vi "探头模板-2-8.vi"() -> ()   [LabVIEW 2017]
uses:
  <vilib>/Utility/miscctls.llb/LVPoint32TypeDef.ctl
  <vilib>/Utility/miscctls.llb/LVPositionTypeDef.ctl
panel:
  in  "鼠标坐标":T1 caption="坐标"
  out "计算时间":dbl
  in  "坐标映射信号":bool=TRUE
  in  "停止":bool=TRUE
  out "探头地址":T2(ring)
  out "探头信息":string
  out "测量值":dbl format="%.2g"
  out "探头状态":T3(ring)=enum."一级报警"
  out "单位":enum16{"μSv/h", "mSv/h"}(ring)
  out "限值1":string="一级限值："
  out "限值2":string="二级限值："
  out "累积剂量":string="二级限值："
  in  "数据簇":T4
  out "数值":string
  in  "XY图":cluster{timestamp[], dbl[]}[](graph)
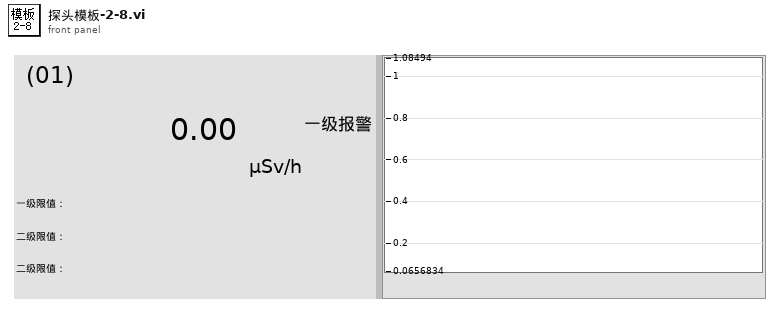
[diagram p1: front panel]
types:
  T1 = typedef "LVPoint32TypeDef.ctl" = cluster{"Horizontal":i32, "Vertical":i32}
  T2 = enum16{"(01)", "(02)", "(03)", "(04)", "(05)", "(06)", "(07)", "(08)", "(09)", "(10)", "(11)", "(12)", "(13)", "(14)", "(15)", "(16)", "(17)", "(18)", "(19)", "(20)", "(21)", "(22)", "(23)", "(24)", "(25)", "(26)", "(27)", "(28)", "(29)", "(30)", "(31)", "(32)", "(33)", "(34)", "(35)"}
  T3 = enum16{"正常", "未启用", "离线", "一级报警", "二级报警", "累积报警"}
  T4 = cluster{"启用状态？":bool, "测量值":cluster{"X":timestamp, "Y":dbl}, "限值簇":cluster{"限值1":dbl, "限值2":dbl, "探头限值":enum16{"一级限值", "二级限值"}}, "报警状态":enum16{"正常", "一级报警", "二级报警", "累积报警"}, "探头信息":string, "探头地址":i32, "累积剂量":cluster{"设备名称":string, "启用累积？":bool, "起始时间":timestamp, "累积剂量":dbl, "累积报警阈值":dbl}}
  T5 = cluster{"限值1":dbl, "限值2":dbl, "探头限值":enum16{"一级限值", "二级限值"}}
  T6 = typedef "LVPositionTypeDef.ctl" = cluster{"Left":i32, "Top":i32}
  T7 = cluster{"设备名称":string, "启用累积？":bool, "起始时间":timestamp, "累积剂量":dbl, "累积报警阈值":dbl}
  T8 = typedef "LVBoundsTypeDef.ctl" = cluster{"Width":u32, "Height":u32}
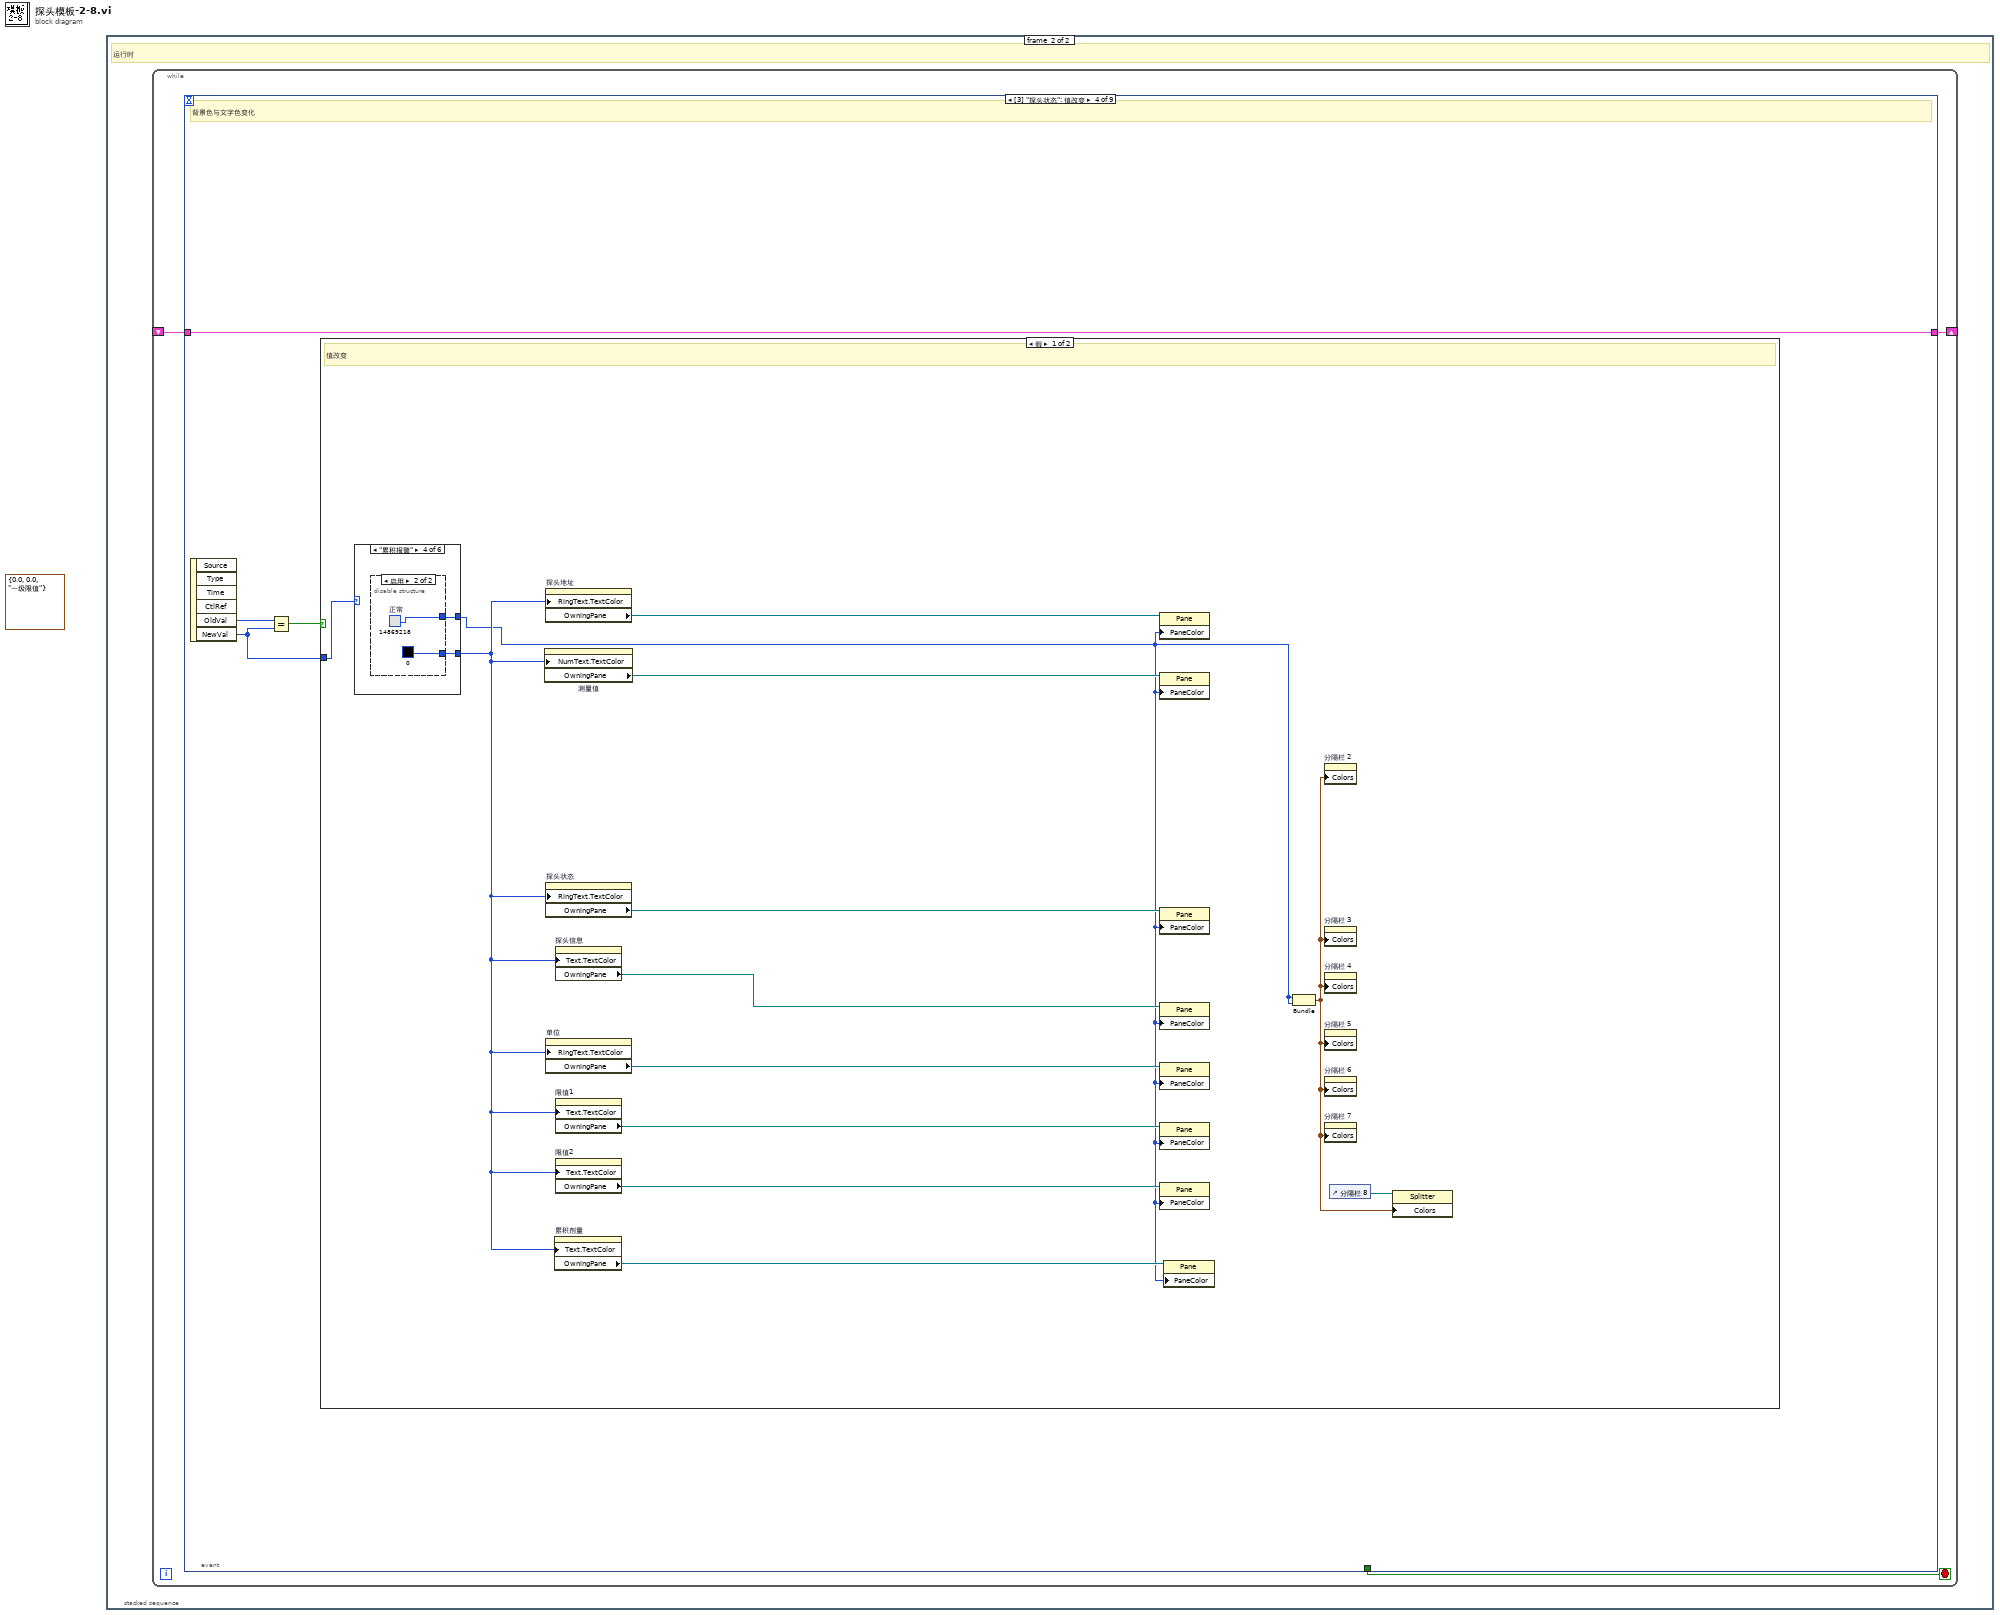
[diagram p0: block diagram]
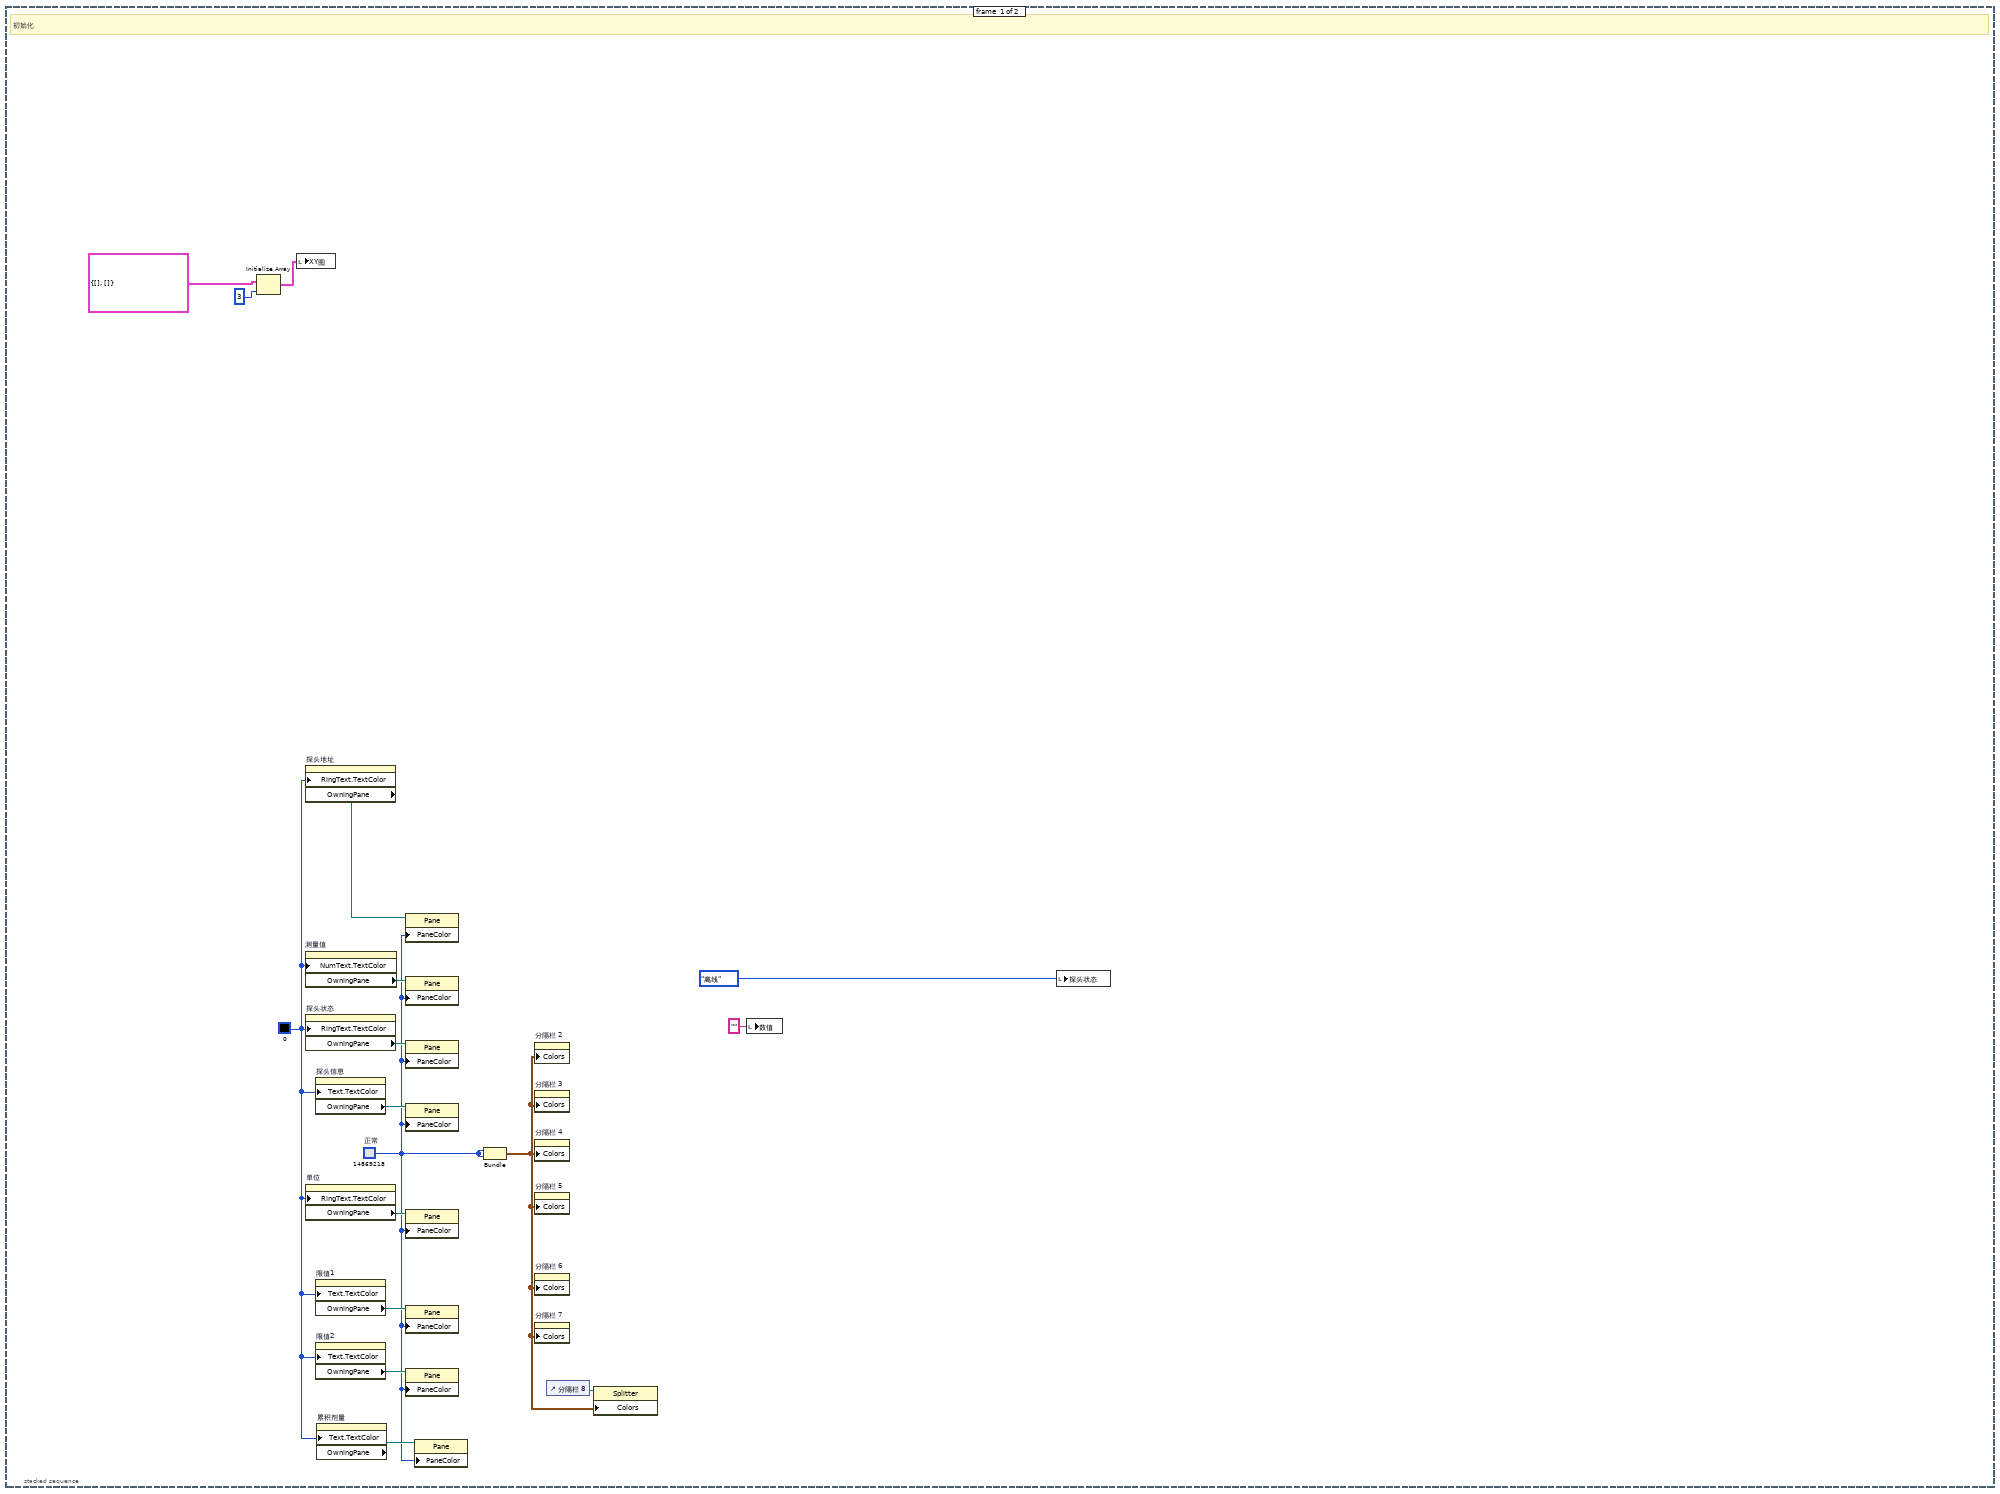
[diagram p2: hidden frame]
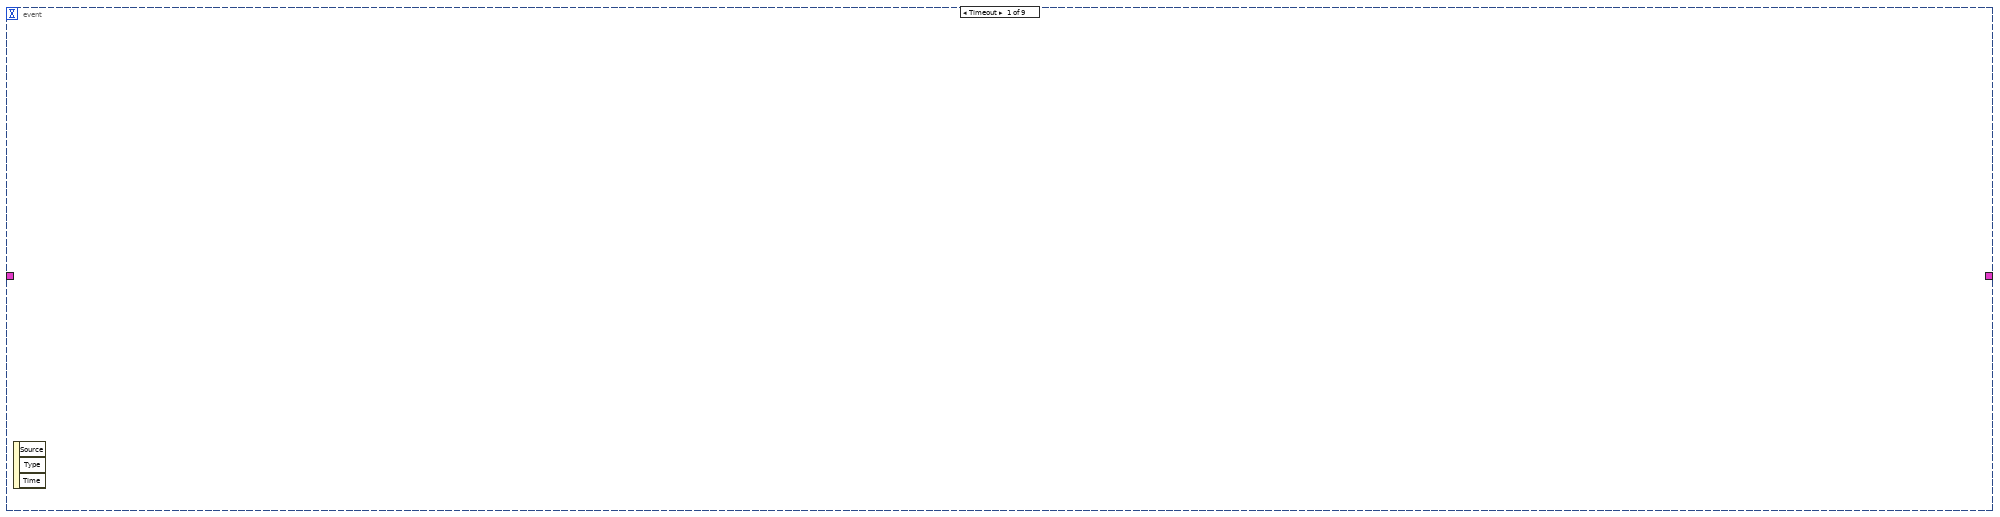
[diagram p3: hidden frame]
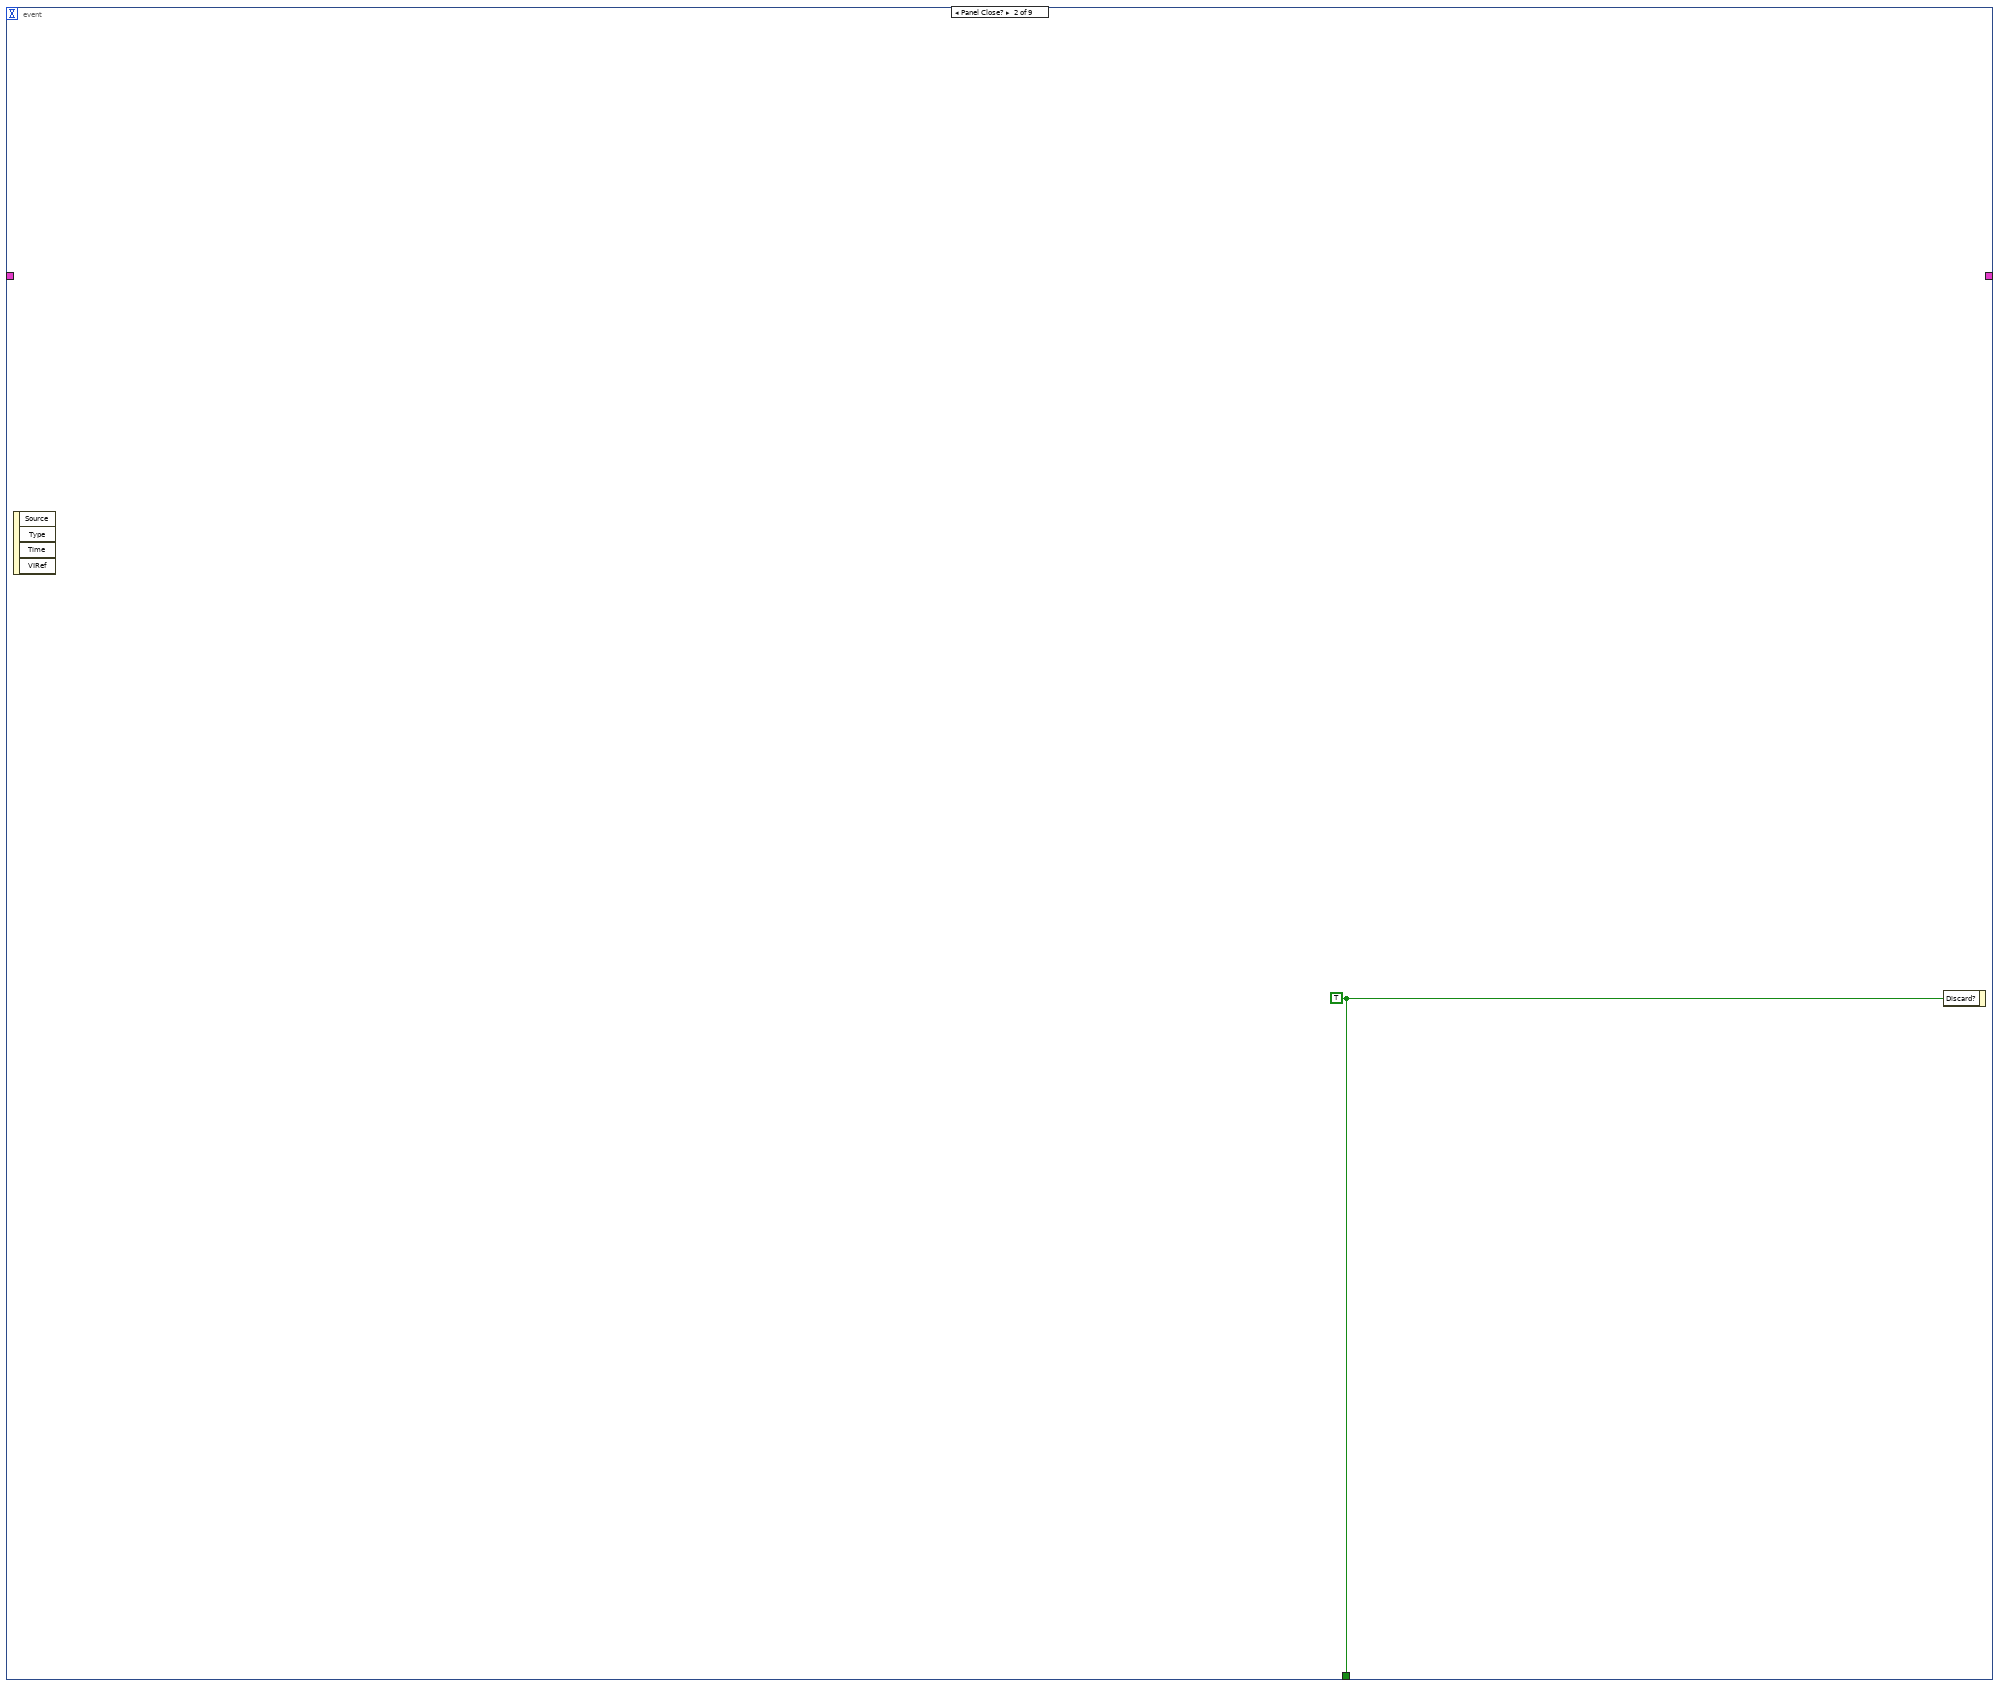
[diagram p4: hidden frame]
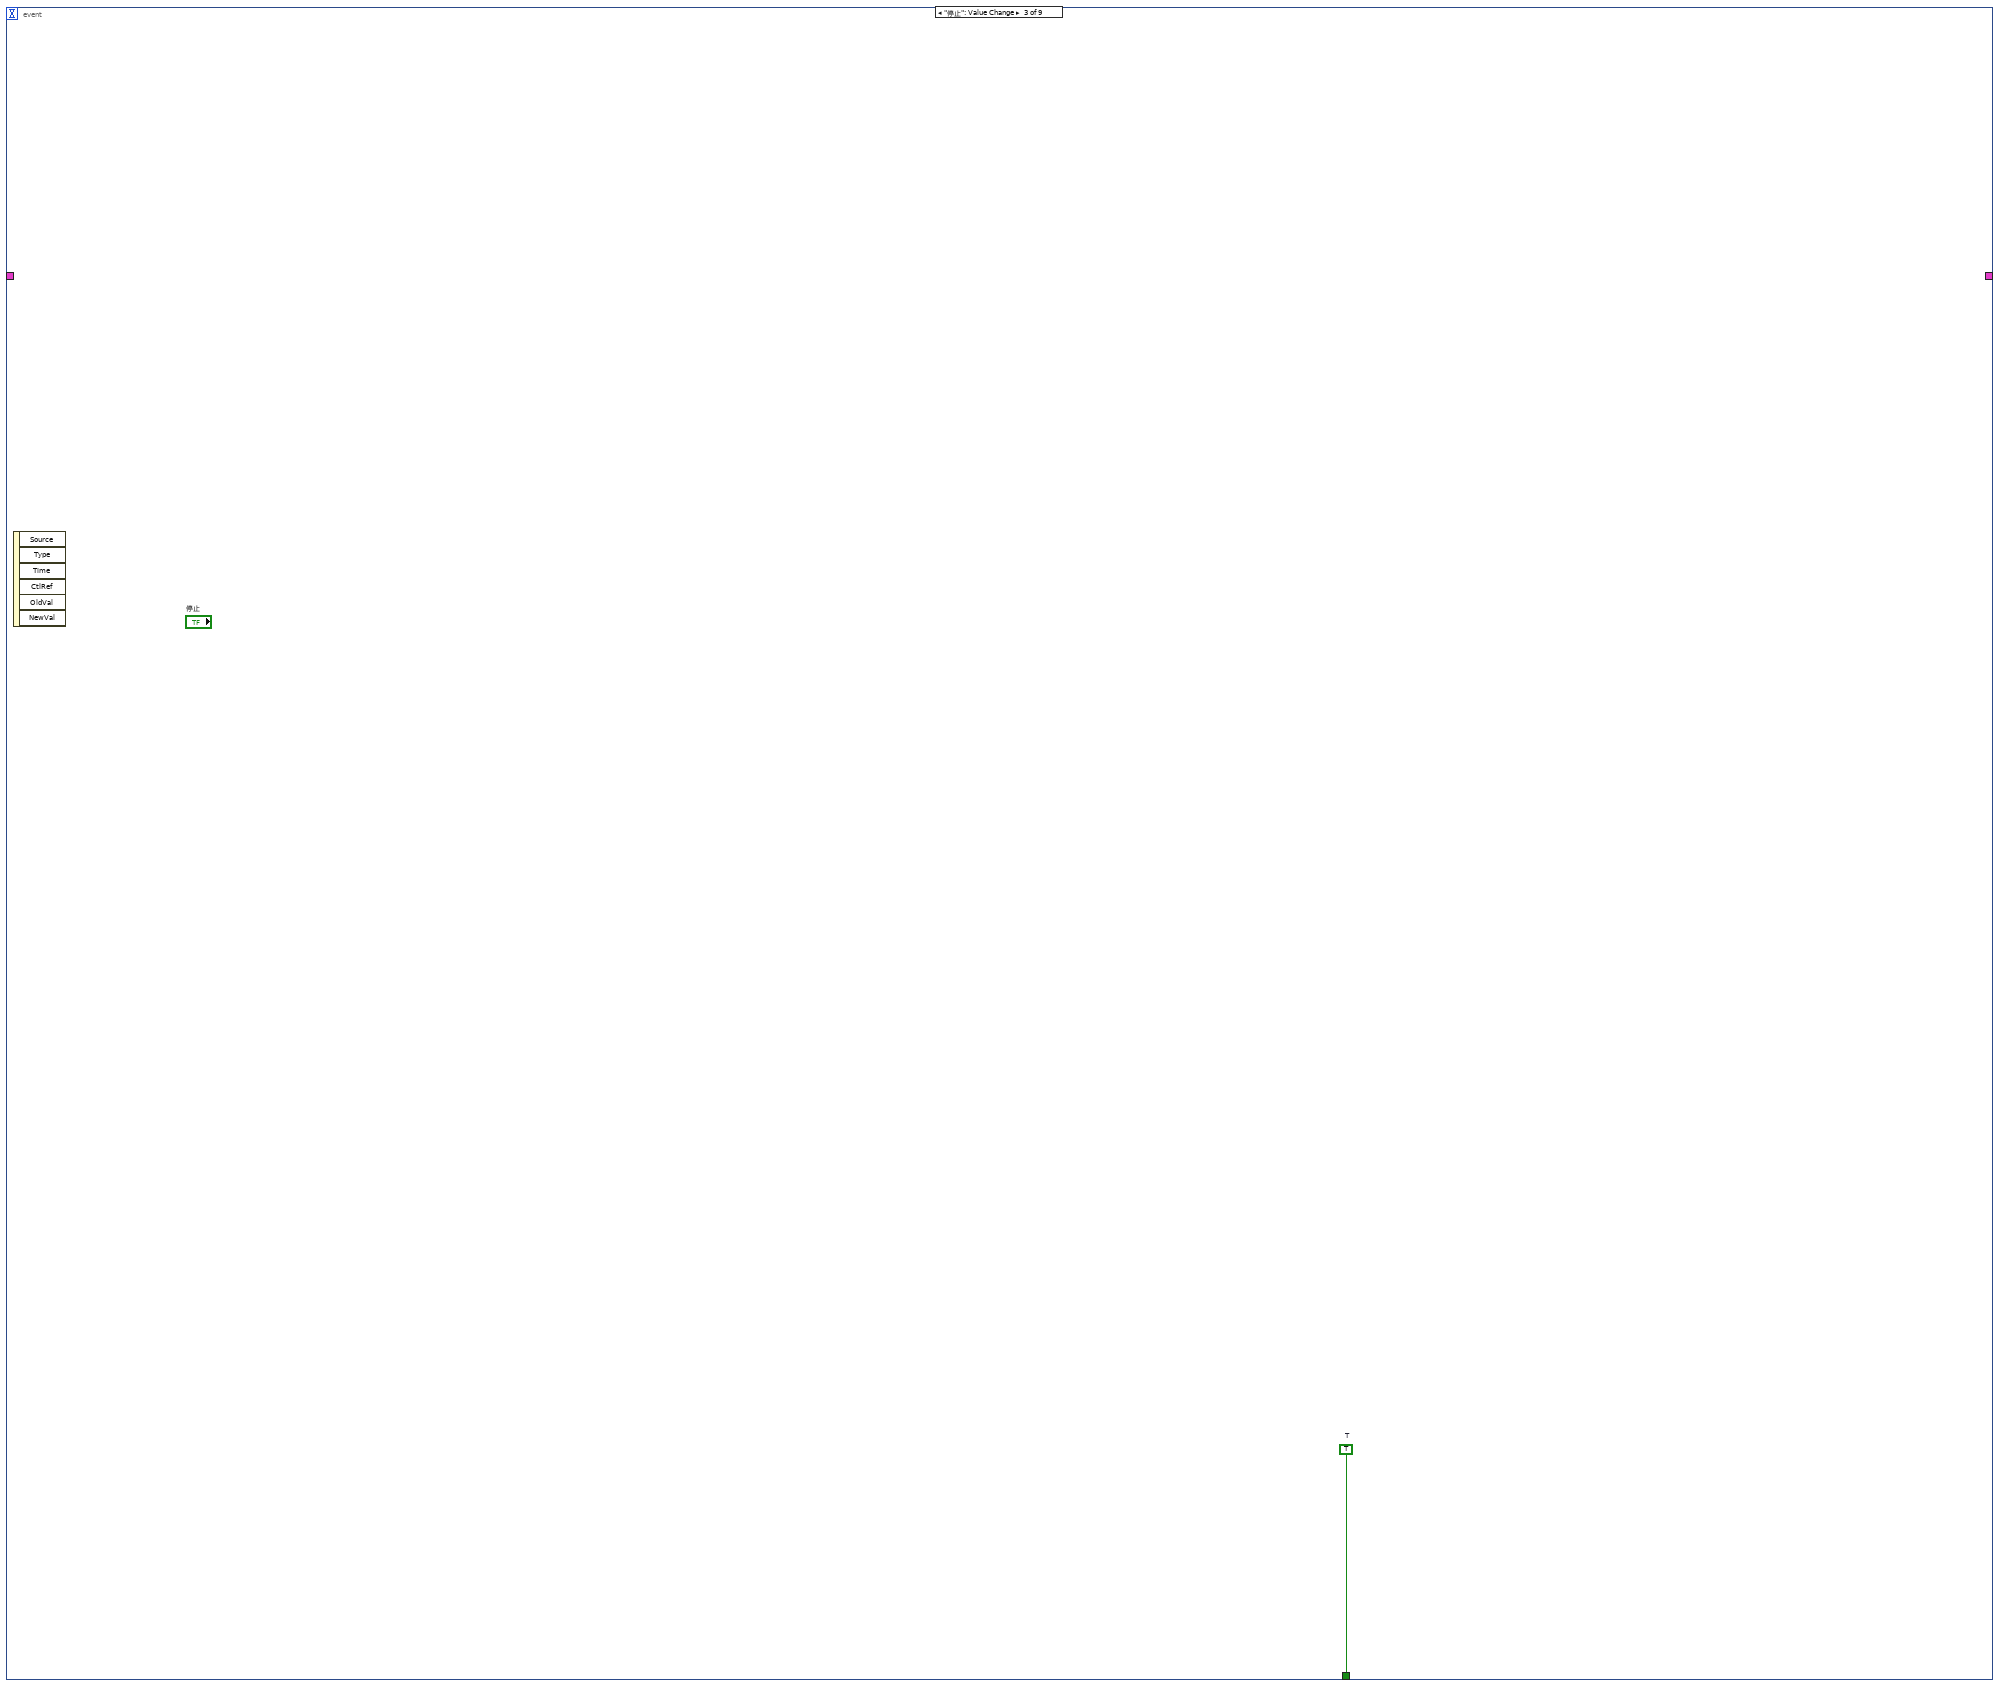
[diagram p5: hidden frame]
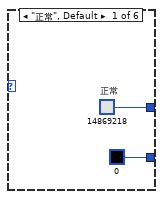
[diagram p6: hidden frame]
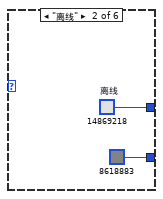
[diagram p7: hidden frame]
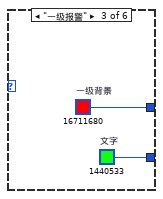
[diagram p8: hidden frame]
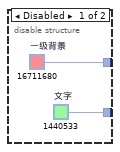
[diagram p9: hidden frame]
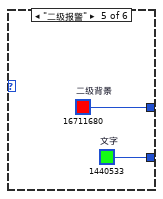
[diagram p10: hidden frame]
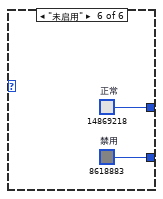
[diagram p11: hidden frame]
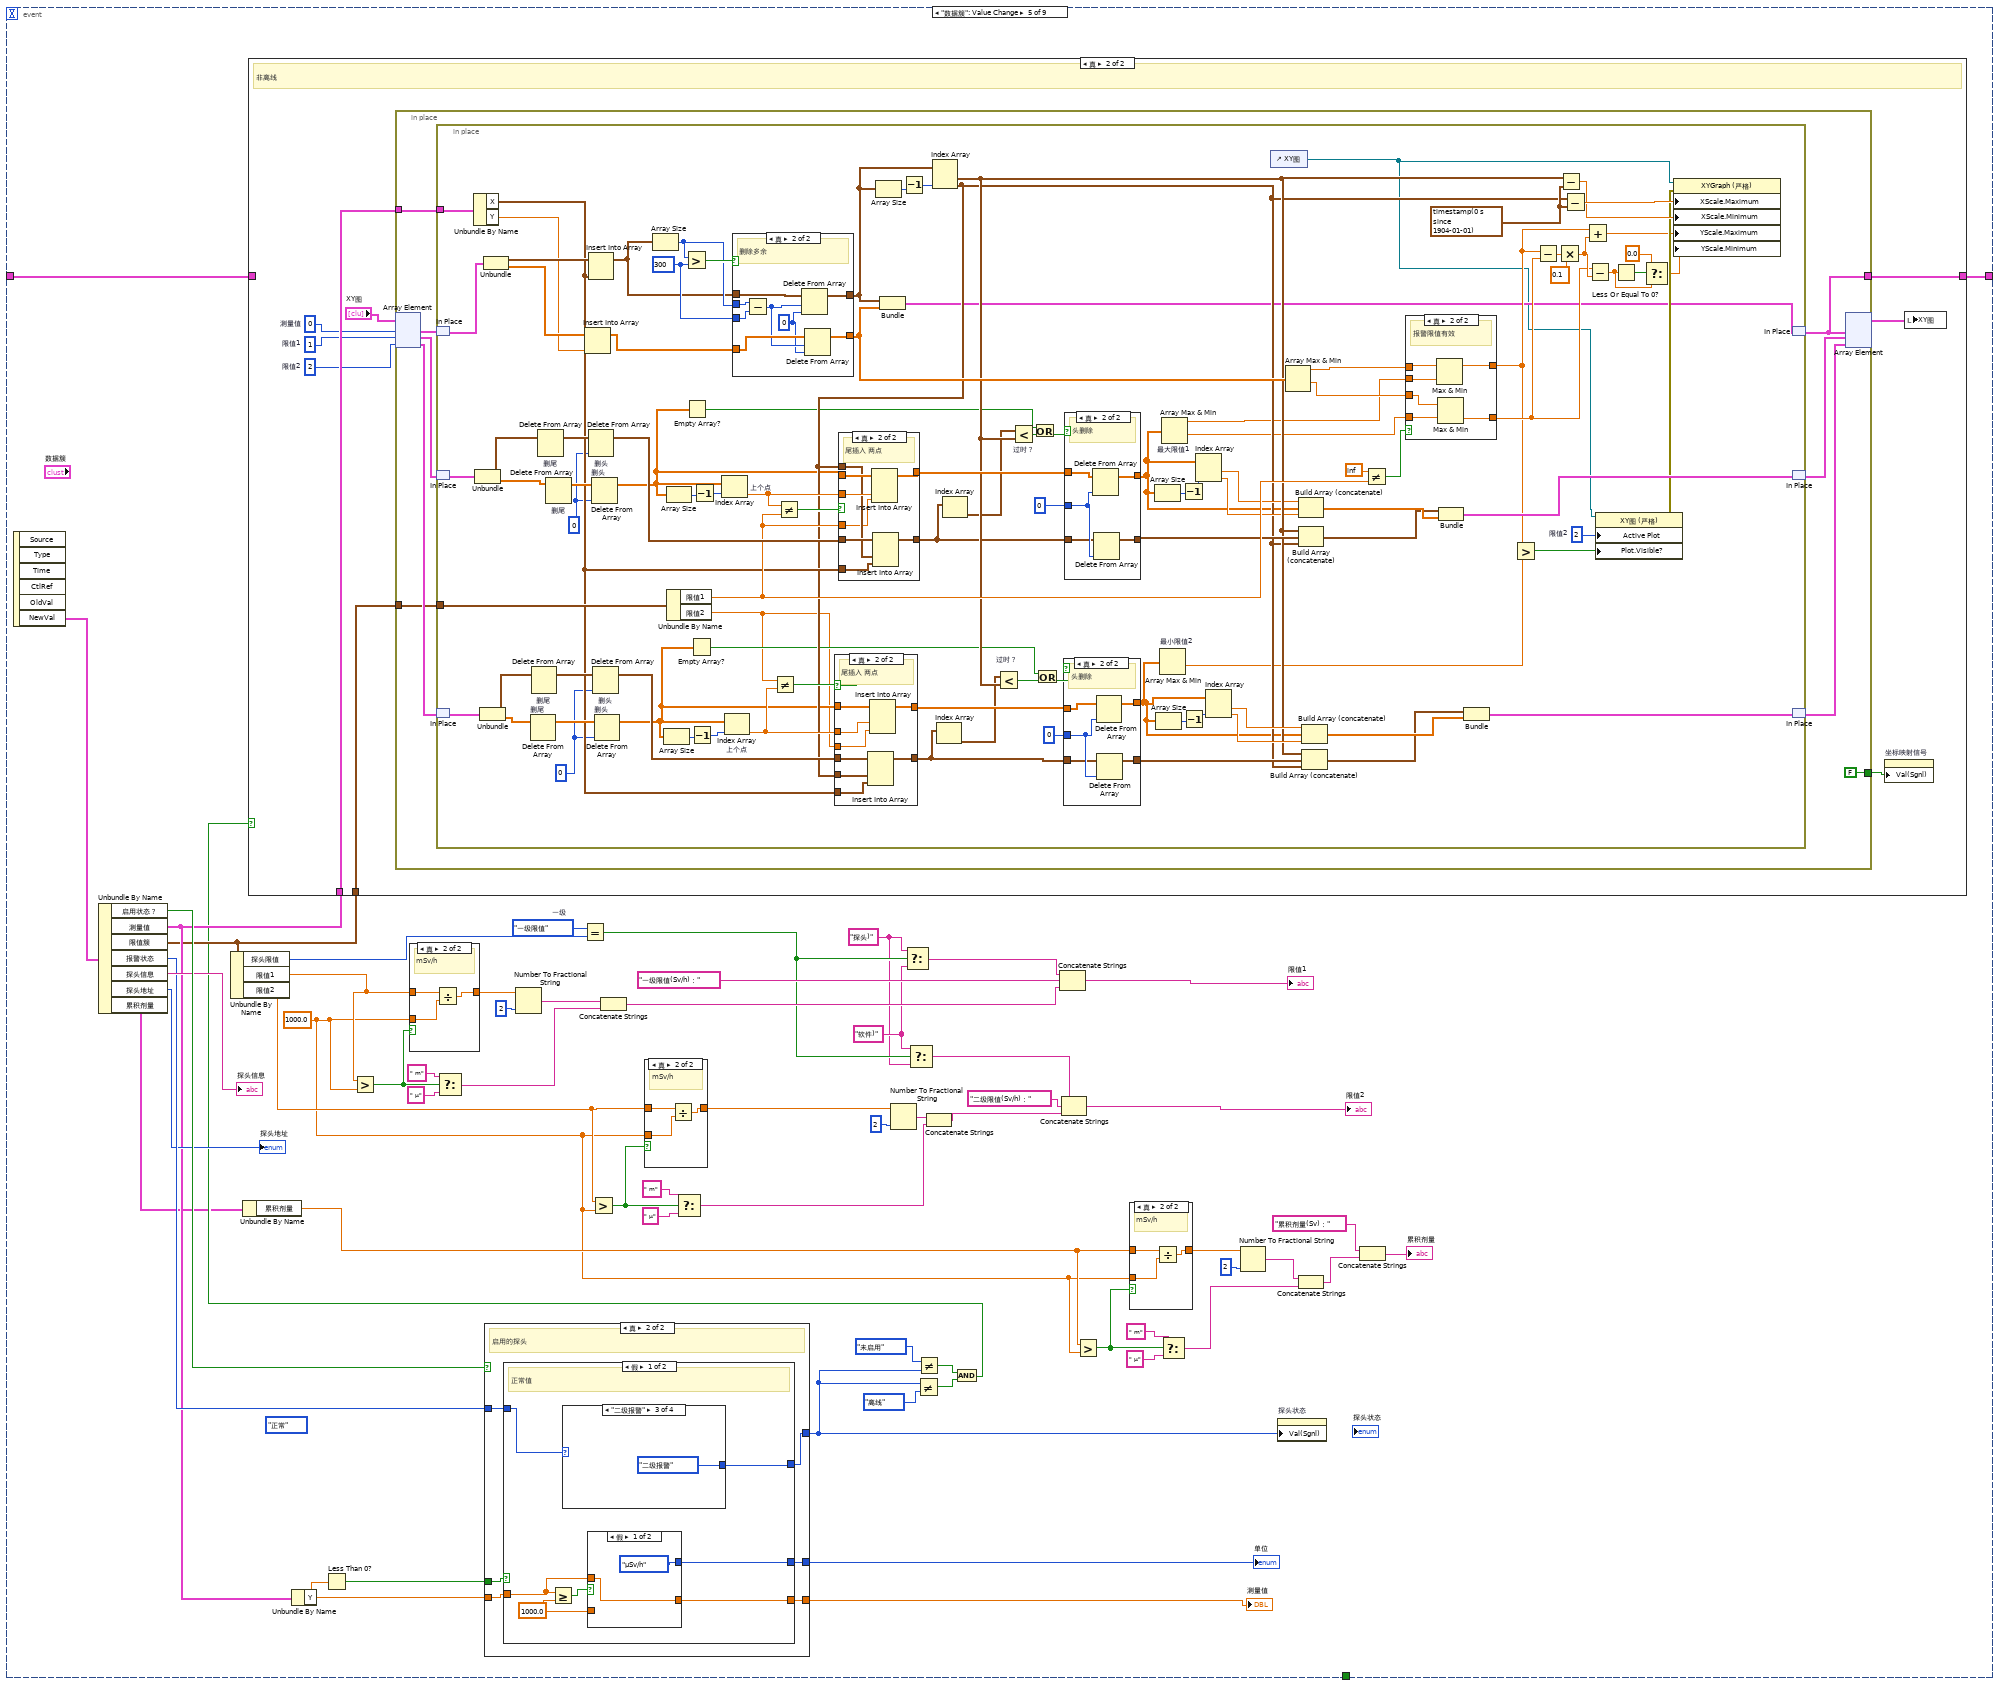
[diagram p13: hidden frame]
diagram:
  (unwired) T5 {"限值1"=0.0, "限值2"=0.0, "探头限值"=enum."一级限值"} ("探头限值簇")
  n1 = stacked-sequence {
    frame #0 {
      w3 = u32 0
      w2 = u32 14869218  # 正常
      # "初始化"
      n2 = Initialize Array(cluster{timestamp[], dbl[]} {[], []}, 3 ("维数大小")) -> (w7:cluster{timestamp[], dbl[]}[])
      n3 = local write "XY图"(w7) -> ()
      n4 = property on="测量值" class="DigNum (严格)"("NumText.TextColor"=w3) -> ("OwningPane"=w16:refnum<vi>)  [unwired: 2 in, 2 out]
      n5 = property on="探头地址" class="Enum (严格)"("RingText.TextColor"=w3) -> ("OwningPane"=w17:refnum<vi>)  [unwired: 2 in, 2 out]
      n6 = property on="探头状态" class="Enum (严格)"("RingText.TextColor"=w3) -> ("OwningPane"=w15:refnum<vi>)  [unwired: 2 in, 2 out]
      n7 = property on="单位" class="Enum (严格)"("RingText.TextColor"=w3) -> ("OwningPane"=w13:refnum<vi>)  [unwired: 2 in, 2 out]
      n8 = property on="探头信息" class="Str"("Text.TextColor"=w3) -> ("OwningPane"=w14:refnum<vi>)  [unwired: 2 in, 2 out]
      n9 = property on="限值1" class="Str"("Text.TextColor"=w3) -> ("OwningPane"=w12:refnum<vi>)  [unwired: 2 in, 2 out]
      n10 = property on="限值2" class="Str"("Text.TextColor"=w3) -> ("OwningPane"=w11:refnum<vi>)  [unwired: 2 in, 2 out]
      n11 = property on="累积剂量" class="Str"("Text.TextColor"=w3) -> ("OwningPane"=w5:refnum<vi>)  [unwired: 2 in, 2 out]
      n12 = property class="Pane"(reference=w17, "PaneColor"=w2) -> ()  [unwired: 1 in, 2 out]
      n13 = property class="Pane"(reference=w16, "PaneColor"=w2) -> ()  [unwired: 1 in, 2 out]
      n14 = property class="Pane"(reference=w15, "PaneColor"=w2) -> ()  [unwired: 1 in, 2 out]
      n15 = property class="Pane"(reference=w14, "PaneColor"=w2) -> ()  [unwired: 1 in, 2 out]
      n16 = property class="Pane"(reference=w13, "PaneColor"=w2) -> ()  [unwired: 1 in, 2 out]
      n17 = property class="Pane"(reference=w12, "PaneColor"=w2) -> ()  [unwired: 1 in, 2 out]
      n18 = property class="Pane"(reference=w11, "PaneColor"=w2) -> ()  [unwired: 1 in, 2 out]
      n19 = property class="Pane"(reference=w5, "PaneColor"=w2) -> ()  [unwired: 1 in, 2 out]
      n20 = Bundle("正常"=w2, "正常"=w2) -> (w1:cluster{"正常":u32, "正常":u32})  [unwired: 1 in]
      n21 = property on="分隔栏 2" class="Splitter"("Colors"=w1) -> ()  [unwired: 2 in, 2 out]
      n22 = property on="分隔栏 3" class="Splitter"("Colors"=w1) -> ()  [unwired: 2 in, 2 out]
      n23 = property on="分隔栏 4" class="Splitter"("Colors"=w1) -> ()  [unwired: 2 in, 2 out]
      n24 = property on="分隔栏 5" class="Splitter"("Colors"=w1) -> ()  [unwired: 2 in, 2 out]
      n25 = property on="分隔栏 6" class="Splitter"("Colors"=w1) -> ()  [unwired: 2 in, 2 out]
      n26 = property on="分隔栏 7" class="Splitter"("Colors"=w1) -> ()  [unwired: 2 in, 2 out]
      n27 = control-ref of="分隔栏 8"() -> (w4:refnum<vi>)
      n28 = property on="属性节点" class="Splitter"(reference=w4, "Colors"=w1) -> ()  [unwired: 1 in, 2 out]
      n29 = local write "数值"("" ("数值")) -> ()
      n30 = local write "探头状态"(enum16{"正常", "未启用", "离线", "一级报警", "二级报警"}."离线" ("探头状态")) -> ()
    }
    frame #1 {
      # "运行时"
      n31 = while {
        shift-right: [w19] -> _
        shift-left: _ -> [w18]
        stop <- w20 stop-if-true
        n32 = event shown="[3] \"探头状态\": 值改变" {
          selector: _ -> [_ _ _ _ _ _ _ _ _]
          dyn-events: _ -> [_ _ _ _ _ _ _ _ _]
          timeout: _ -> [_ _ _ _ _ _ _ _ _]
          tunnel: [_ w21 w22 _ _ _ _ _ _] -> w20
          tunnel: [_ _ _ w23 w83 w326 w380 w382 w384] -> w19
          tunnel: w18 -> [_ _ _ w23 w76 w326 w380 w382 w384]
          event Timeout {
            n33 = event-data() -> ()  [unwired: 1 in, 3 out]
          }
          event Panel Close? {
            w21 = TRUE ("放弃？")
            n34 = event-data() -> ()  [unwired: 1 in, 4 out]
            n35 = event-data("Discard?"=w21) -> ()  [unwired: 1 in, 1 out]
          }
          event "停止": Value Change {
            w22 = TRUE  # T
            n36 = event-data() -> ()  [unwired: 1 in, 6 out]
          }
          event "探头状态": Value Change {
            # "背景色与文字色变化"
            n37 = event-data() -> ("OldVal"=w26:T3, "NewVal"=w25:T3)  [unwired: 1 in, 4 out]
            n38 = Equal?(x=w26, y=w25) -> (x = y?=w24:bool)
            n39 = case shown="假" w24 {
              tunnel: w25 -> [w39 _]
              frame False {
                # "值改变"
                n40 = case shown="\"累积报警\"" w39 {
                  tunnel: [w40 w42 w45 w47 w53 w54] -> w29
                  tunnel: [u32 0 u32 8618883 w44 w46 w52 w55] -> w31
                  frame "正常", Default {
                    w40 = u32 14869218  # 正常
                  }
                  frame "离线" {
                    w42 = u32 14869218  # 离线
                  }
                  frame "一级报警" {
                    w44 = u32 1440533  # 文字
                    w45 = u32 16711680  # 一级背景
                  }
                  frame "累积报警" {
                    n41 = disable-structure shown="启用" {
                      disable-tunnel: [w49 w51] -> w47
                      disable-tunnel: [w48 u32 0] -> w46
                      frame Disabled {
                        w48 = u32 1440533  # 文字
                        w49 = u32 16711680  # 一级背景
                      }
                      frame Enabled {
                        w51 = u32 14869218  # 正常
                      }
                    }
                  }
                  frame "二级报警" {
                    w52 = u32 1440533  # 文字
                    w53 = u32 16711680  # 二级背景
                  }
                  frame "未启用" {
                    w54 = u32 14869218  # 正常
                    w55 = u32 8618883  # 禁用
                  }
                }
                n42 = property on="测量值" class="DigNum (严格)"("NumText.TextColor"=w31) -> ("OwningPane"=w37:refnum<vi>)  [unwired: 2 in, 2 out]
                n43 = property on="探头地址" class="Enum (严格)"("RingText.TextColor"=w31) -> ("OwningPane"=w38:refnum<vi>)  [unwired: 2 in, 2 out]
                n44 = property on="探头状态" class="Enum (严格)"("RingText.TextColor"=w31) -> ("OwningPane"=w36:refnum<vi>)  [unwired: 2 in, 2 out]
                n45 = property on="单位" class="Enum (严格)"("RingText.TextColor"=w31) -> ("OwningPane"=w34:refnum<vi>)  [unwired: 2 in, 2 out]
                n46 = property on="累积剂量" class="Str"("Text.TextColor"=w31) -> ("OwningPane"=w30:refnum<vi>)  [unwired: 2 in, 2 out]
                n47 = property on="探头信息" class="Str"("Text.TextColor"=w31) -> ("OwningPane"=w35:refnum<vi>)  [unwired: 2 in, 2 out]
                n48 = property on="限值1" class="Str"("Text.TextColor"=w31) -> ("OwningPane"=w33:refnum<vi>)  [unwired: 2 in, 2 out]
                n49 = property on="限值2" class="Str"("Text.TextColor"=w31) -> ("OwningPane"=w32:refnum<vi>)  [unwired: 2 in, 2 out]
                n50 = property class="Pane"(reference=w38, "PaneColor"=w29) -> ()  [unwired: 1 in, 2 out]
                n51 = property class="Pane"(reference=w37, "PaneColor"=w29) -> ()  [unwired: 1 in, 2 out]
                n52 = property class="Pane"(reference=w36, "PaneColor"=w29) -> ()  [unwired: 1 in, 2 out]
                n53 = property class="Pane"(reference=w35, "PaneColor"=w29) -> ()  [unwired: 1 in, 2 out]
                n54 = property class="Pane"(reference=w34, "PaneColor"=w29) -> ()  [unwired: 1 in, 2 out]
                n55 = property class="Pane"(reference=w33, "PaneColor"=w29) -> ()  [unwired: 1 in, 2 out]
                n56 = property class="Pane"(reference=w32, "PaneColor"=w29) -> ()  [unwired: 1 in, 2 out]
                n57 = property class="Pane"(reference=w30, "PaneColor"=w29) -> ()  [unwired: 1 in, 2 out]
                n58 = Bundle("正常"=w29, "正常"=w29) -> (w27:cluster{"正常":u32, "正常":u32})  [unwired: 1 in]
                n59 = property on="分隔栏 2" class="Splitter"("Colors"=w27) -> ()  [unwired: 2 in, 2 out]
                n60 = property on="分隔栏 3" class="Splitter"("Colors"=w27) -> ()  [unwired: 2 in, 2 out]
                n61 = property on="分隔栏 4" class="Splitter"("Colors"=w27) -> ()  [unwired: 2 in, 2 out]
                n62 = property on="分隔栏 5" class="Splitter"("Colors"=w27) -> ()  [unwired: 2 in, 2 out]
                n63 = property on="分隔栏 6" class="Splitter"("Colors"=w27) -> ()  [unwired: 2 in, 2 out]
                n64 = property on="分隔栏 7" class="Splitter"("Colors"=w27) -> ()  [unwired: 2 in, 2 out]
                n65 = control-ref of="分隔栏 8"() -> (w28:refnum<vi>)
                n66 = property on="属性节点" class="Splitter"(reference=w28, "Colors"=w27) -> ()  [unwired: 1 in, 2 out]
              }
              frame True {
              }
            }
          }
          event "数据簇": Value Change {
            w58 = "软件)" ("字符串")
            w57 = "探头)" ("字符串")
            w61 = enum16{"一级限值", "二级限值"}."一级限值"  # 一级
            (unwired) enum16{"正常", "一级报警", "二级报警", "累积报警"}."正常" ("报警状态")
            w69 = 1000.0 ("y")
            n67 = event-data() -> ("NewVal"=w116:T4)  [unwired: 1 in, 5 out]
            n68 = Unbundle By Name(w116) -> ("启用状态？"=w111:bool, "测量值"=w85:cluster{"X":timestamp, "Y":dbl}, "限值簇"=w84:T5, "报警状态"=w105:enum16{"正常", "一级报警", "二级报警", "累积报警"}, "探头信息"=→"探头信息":string, "探头地址"=→"探头地址":i32, "累积剂量"=w75:T7)
            n69 = Unbundle By Name(w84) -> ("探头限值"=w62:enum16{"一级限值", "二级限值"}, "限值1"=w89:dbl, "限值2"=w87:dbl)
            n70 = Unbundle By Name(w75) -> ("累积剂量"=w70:dbl)
            n71 = Unbundle By Name(w85) -> ("Y"=w109:dbl)
            n72 = Less Than 0?(x=w109) -> (x < 0?=w110:bool)
            n73 = Greater?(x=w89, y=w69) -> (0:w102:bool)
            n74 = case shown="真" w102 {
              tunnel: w89 -> [w297 w300]
              tunnel: w69 -> [_ w299]
              tunnel: [w297 w298] -> w97
              frame False {
                # "uSv/h"
              }
              frame True {
                # "mSv/h"
                n75 = Divide(x=w300, y=w299) -> (x/y=w298:dbl)
              }
            }
            n76 = Select(t=" m" ("F-格式字符串"), s=w102, f=" μ" ("F-格式字符串")) -> (s? t:f=w98:string)
            n77 = case shown="真" w111 {
              tunnel: w110 -> [_ w307]
              tunnel: w109 -> [_ w306]
              tunnel: [_ w305] -> w107
              tunnel: [_ w304] -> w108
              tunnel: [enum16{"正常", "未启用", "离线", "一级报警", "二级报警"}."未启用" ("探头状态") w303] -> w82
              tunnel: w105 -> [_ w302]
              frame False {
                # "未启用的探头"
              }
              frame True {
                # "启用的探头"
                n78 = case shown="假" w307 {
                  tunnel: w306 -> [w313 _]
                  tunnel: [w311 _] -> w305
                  tunnel: [w310 _] -> w304
                  tunnel: [w308 enum16{"正常", "未启用", "离线", "一级报警", "二级报警"}."离线" ("探头状态")] -> w303
                  tunnel: w302 -> [w309 _]
                  frame False {
                    w312 = 1000.0 ("y")
                    # "正常值"
                    n79 = Greater Or Equal?(x=w313, y=w312) -> (x >= y?=w314:bool)
                    n80 = case shown="\"二级报警\"" w309 {
                      tunnel: [enum16{"正常", "未启用", "离线", "一级报警", "二级报警"}."正常" ("探头状态") enum16{"正常", "未启用", "离线", "一级报警", "二级报警"}."一级报警" ("探头状态") enum16{"正常", "未启用", "离线", "一级报警", "二级报警"}."二级报警" ("探头状态") T3."累积报警" ("探头状态")] -> w308
                      frame "正常", Default {
                      }
                      frame "一级报警" {
                      }
                      frame "二级报警" {
                      }
                      frame "累积报警" {
                      }
                    }
                    n81 = case shown="假" w314 {
                      tunnel: w313 -> [w320 w324]
                      tunnel: w312 -> [_ w323]
                      tunnel: [w320 w322] -> w311
                      tunnel: [enum16{"μSv/h", "mSv/h"}."μSv/h" ("单位") enum16{"μSv/h", "mSv/h"}."mSv/h" ("单位")] -> w310
                      frame False {
                      }
                      frame True {
                        n82 = Divide(x=w324, y=w323) -> (x/y=w322:dbl)
                      }
                    }
                  }
                  frame True {
                    # "掉线"
                  }
                }
              }
            }
            "单位" <- w108
            "测量值" <- w107
            n83 = Number To Fractional String(number=w97, precision (6)=i16 2 ("精度(6)")) -> (F-format string=w101:string)  [unwired: 2 in]
            n84 = Equal?(x=w61, y=w62) -> (x = y?=w60:bool)
            n85 = Greater?(x=w87, y=w69) -> (0:w95:bool)
            n86 = Concatenate Strings(w101, w98) -> (w88:string)
            n87 = case shown="真" w95 {
              tunnel: w87 -> [w293 w296]
              tunnel: w69 -> [_ w295]
              tunnel: [w293 w294] -> w90
              frame False {
                # "uSv/h"
              }
              frame True {
                # "mSv/h"
                n88 = Divide(x=w296, y=w295) -> (x/y=w294:dbl)
              }
            }
            n89 = Select(t=" m" ("F-格式字符串"), s=w95, f=" μ" ("F-格式字符串")) -> (s? t:f=w91:string)
            n90 = Number To Fractional String(number=w90, precision (6)=i16 2 ("精度(6)")) -> (F-format string=w94:string)  [unwired: 2 in]
            n91 = Select(t=w57, s=w60, f=w58) -> (s? t:f=w59:string)
            n92 = Select(t=w58, s=w60, f=w57) -> (s? t:f=w56:string)
            n93 = Not Equal?(x=w82, y=enum16{"正常", "未启用", "离线", "一级报警", "二级报警"}."离线" ("探头状态")) -> (x != y?=w79:bool)
            n94 = Not Equal?(x=enum16{"正常", "未启用", "离线", "一级报警", "二级报警"}."未启用" ("探头状态"), y=w82) -> (x != y?=w78:bool)
            n95 = Concatenate Strings(w94, w91) -> (w86:string)
            n96 = And(x=w78, y=w79) -> (x .and. y?=w77:bool)
            n97 = case shown="真" w77 {
              tunnel: w85 -> [_ w130]
              tunnel: w84 -> [_ w125]
              tunnel: [w121 w123] -> w83
              tunnel: w76 -> [w121 _]
              frame False {
                # "离线不更新曲线"
              }
              frame True {
                w126 = 2  # 限值2
                w127 = 1  # 限值1
                w128 = 0  # 测量值
                # "非离线"
                n98 = in-place {
                  in-place-border: w130 -> [w139]
                  in-place-border: w125 -> [w135]
                  in-place-border: [w132] -> w123
                  in-place-border: [FALSE ("值(信号)")] -> w122
                  n99 = in-place-array #1("XY图", w128, w127, w126) -> (w138:cluster{timestamp[], dbl[]}, w136:cluster{timestamp[], dbl[]}, w137:cluster{timestamp[], dbl[]})
                  n100 = in-place {
                    in-place-border: w139 -> [w234]
                    in-place-border: w135 -> [w228]
                    w164 = 0 ("索引")
                    w165 = 0 ("索引")
                    w226 = u32 2  # 限值2
                    w235 = 300 ("y")
                    w240 = timestamp(0 s since 1904-01-01)
                    n101 = in-place-match #2(w138) -> (w229:cluster{timestamp[], dbl[]})
                    n102 = in-place-match #3(w136) -> (w194:cluster{timestamp[], dbl[]})
                    n103 = in-place-match #4(w137) -> (w175:cluster{timestamp[], dbl[]})
                    n104 = Unbundle By Name(w234) -> ("X"=w174:timestamp, "Y"=w225:dbl)
                    n105 = Unbundle(w194) -> (w198:timestamp[], w197:dbl[])
                    n106 = Unbundle(w175) -> (w179:timestamp[], w178:dbl[])
                    n107 = Unbundle(w229) -> (w233:timestamp[], w232:dbl[])
                    n108 = Delete From Array "删尾"(array=w178) -> (array with subset deleted=w177:dbl[])  [unwired: 2 in, 1 out]
                    n109 = Delete From Array "删尾"(array=w179) -> (array with subset deleted=w180:timestamp[])  [unwired: 2 in, 1 out]
                    n110 = Delete From Array "删尾"(array=w198) -> (array with subset deleted=w199:timestamp[])  [unwired: 2 in, 1 out]
                    n111 = Delete From Array "删尾"(array=w197) -> (array with subset deleted=w196:dbl[])  [unwired: 2 in, 1 out]
                    n112 = Insert Into Array(array=w232, new element=w225) -> (w230:dbl[])  [unwired: 1 in]
                    n113 = Insert Into Array(array=w233, new element=w174) -> (w231:timestamp[])  [unwired: 1 in]
                    n114 = Delete From Array "删头"(array=w199, index=w165) -> (array with subset deleted=w202:timestamp[])  [unwired: 1 in, 1 out]
                    n115 = Delete From Array "删头"(array=w196, index=w165) -> (array with subset deleted=w153:dbl[])  [unwired: 1 in, 1 out]
                    n116 = Delete From Array "删头"(array=w180, index=w164) -> (array with subset deleted=w184:timestamp[])  [unwired: 1 in, 1 out]
                    n117 = Delete From Array "删头"(array=w177, index=w164) -> (array with subset deleted=w152:dbl[])  [unwired: 1 in, 1 out]
                    n118 = Array Size(array=w231) -> (size(s)=w236:i32)
                    n119 = Array Size(array=w152) -> (size(s)=w181:i32)
                    n120 = Array Size(array=w153) -> (size(s)=w195:i32)
                    n121 = Unbundle By Name(w228) -> ("限值1"=w193:dbl, "限值2"=w147:dbl)
                    n122 = Greater?(x=w236, y=w235) -> (0:w237:bool)
                    n123 = Empty Array?(array=w153) -> (empty?=w151:bool)
                    n124 = Empty Array?(array=w152) -> (empty?=w150:bool)
                    n125 = Decrement(x=w181) -> (x-1=w182:i32)
                    n126 = Decrement(x=w195) -> (x-1=w200:i32)
                    n127 = Index Array "上个点"(array=w153, index=w200) -> (element=w163:dbl)
                    n128 = Index Array "上个点"(array=w152, index=w182) -> (element=w162:dbl)
                    n129 = case shown="真" w237 {
                      tunnel: w231 -> [w284 w292]
                      tunnel: w236 -> [_ w291]
                      tunnel: w235 -> [_ w290]
                      tunnel: [w284 w289] -> w224
                      tunnel: w230 -> [w283 w288]
                      tunnel: [w283 w285] -> w220
                      frame False {
                      }
                      frame True {
                        w286 = 0 ("索引")
                        # "删除多余"
                        n130 = Subtract(x=w291, y=w290) -> (x-y=w287:i32)
                        n131 = Delete From Array(array=w292, length=w287, index=w286) -> (array with subset deleted=w289:timestamp[])  [unwired: 1 out]
                        n132 = Delete From Array(array=w288, length=w287, index=w286) -> (array with subset deleted=w285:dbl[])  [unwired: 1 out]
                      }
                    }
                    n133 = Not Equal?(x=w147, y=w162) -> (x != y?=w176:bool)
                    n134 = Not Equal?(x=w163, y=w193) -> (x != y?=w166:bool)
                    n135 = Array Size(array=w224) -> (size(s)=w223:i32)
                    n136 = Bundle(w224, w220) -> (w141:cluster{timestamp[], dbl[]})  [unwired: 1 in]
                    n137 = Decrement(x=w223) -> (x-1=w222:i32)
                    n138 = Index Array(array=w224, index #2=w222) -> (element #1=w171:timestamp, element #2=w161:timestamp)  [unwired: 1 in]
                    n139 = case shown="真" w176 {
                      tunnel: [w249 w251] -> w160
                      tunnel: w152 -> [w249 w257]
                      tunnel: w147 -> [_ w250]
                      tunnel: w184 -> [w248 w256]
                      tunnel: w174 -> [_ w253]
                      tunnel: [w248 w252] -> w157
                      tunnel: w162 -> [_ w255]
                      tunnel: w161 -> [_ w254]
                      frame False {
                        # "不插入"
                      }
                      frame True {
                        # "尾插入 两点"
                        n140 = Insert Into Array(array=w256, new element #1=w254, new element #2=w253) -> (w252:timestamp[])  [unwired: 1 in]
                        n141 = Insert Into Array(array=w257, new element #1=w255, new element #2=w250) -> (w251:dbl[])  [unwired: 1 in]
                      }
                    }
                    n142 = case shown="真" w166 {
                      tunnel: [w266 w270] -> w203
                      tunnel: w153 -> [w266 w274]
                      tunnel: w193 -> [_ w267]
                      tunnel: w174 -> [_ w268]
                      tunnel: w202 -> [w265 w273]
                      tunnel: [w265 w269] -> w159
                      tunnel: w163 -> [_ w272]
                      tunnel: w161 -> [_ w271]
                      frame False {
                        # "不插入"
                      }
                      frame True {
                        # "尾插入 两点"
                        n143 = Insert Into Array(array=w274, new element #1=w272, new element #2=w267) -> (w270:dbl[])  [unwired: 1 in]
                        n144 = Insert Into Array(array=w273, new element #1=w271, new element #2=w268) -> (w269:timestamp[])  [unwired: 1 in]
                      }
                    }
                    n145 = Index Array(array=w157) -> (element=w156:timestamp)  [unwired: 1 in]
                    n146 = Index Array(array=w159) -> (element=w158:timestamp)  [unwired: 1 in]
                    n147 = Less? "过时？"(x=w156, y=w171) -> (x < y?=w183:bool)
                    n148 = Less? "过时？"(x=w158, y=w171) -> (x < y?=w201:bool)
                    n149 = Or(x=w151, y=w201) -> (x .or. y?=w155:bool)
                    n150 = Or(x=w150, y=w183) -> (x .or. y?=w154:bool)
                    n151 = case shown="真" w154 {
                      tunnel: w160 -> [w242 w246]
                      tunnel: w157 -> [w241 w245]
                      tunnel: 0 ("索引") -> [_ w247]
                      tunnel: [w242 w244] -> w149
                      tunnel: [w241 w243] -> w188
                      frame False {
                      }
                      frame True {
                        # "头删除"
                        n152 = Delete From Array(array=w246, index=w247) -> (array with subset deleted=w244:dbl[])  [unwired: 1 in, 1 out]
                        n153 = Delete From Array(array=w245, index=w247) -> (array with subset deleted=w243:timestamp[])  [unwired: 1 in, 1 out]
                      }
                    }
                    n154 = case shown="真" w155 {
                      tunnel: w203 -> [w259 w264]
                      tunnel: w159 -> [w258 w262]
                      tunnel: 0 ("索引") -> [_ w263]
                      tunnel: [w259 w261] -> w148
                      tunnel: [w258 w260] -> w172
                      frame False {
                      }
                      frame True {
                        # "头删除"
                        n155 = Delete From Array(array=w264, index=w263) -> (array with subset deleted=w261:dbl[])  [unwired: 1 in, 1 out]
                        n156 = Delete From Array(array=w262, index=w263) -> (array with subset deleted=w260:timestamp[])  [unwired: 1 in, 1 out]
                      }
                    }
                    n157 = Array Size(array=w148) -> (size(s)=w205:i32)
                    n158 = Array Size(array=w149) -> (size(s)=w187:i32)
                    n159 = Array Max & Min "最小限值2"(array=w149) -> (min value=w143:dbl)  [unwired: 3 out]
                    n160 = Array Max & Min "最大限值1"(array=w148) -> (max value=w146:dbl, min value=w145:dbl)  [unwired: 2 out]
                    n161 = Decrement(x=w205) -> (x-1=w206:i32)
                    n162 = Decrement(x=w187) -> (x-1=w186:i32)
                    n163 = Index Array(array=w148, index #2=w206) -> (element #1=w170:dbl, element #2=w169:dbl)  [unwired: 1 in]
                    n164 = Index Array(array=w149, index #2=w186) -> (element #1=w189:dbl, element #2=w190:dbl)  [unwired: 1 in]
                    n165 = control-ref of="XY图"() -> (w140:refnum<vi>)
                    n166 = Array Max & Min(array=w220) -> (max value=w211:dbl, min value=w210:dbl)  [unwired: 2 out]
                    n167 = Build Array (concatenate)(w170, w148, w169) -> (w168:dbl[])
                    n168 = Build Array (concatenate)(w171, w172, w161) -> (w167:timestamp[])
                    n169 = Build Array (concatenate)(w189, w149, w190) -> (w192:dbl[])
                    n170 = Build Array (concatenate)(w171, w188, w161) -> (w191:timestamp[])
                    n171 = Not Equal?(x=inf, y=w193) -> (x != y?=w208:bool)
                    n172 = case shown="真" w208 {
                      tunnel: w211 -> [w276 w282]
                      tunnel: [w276 w281] -> w144
                      tunnel: w145 -> [_ w280]
                      tunnel: w210 -> [w275 w279]
                      tunnel: [w275 w278] -> w209
                      tunnel: w146 -> [_ w277]
                      frame False {
                        # "报警限值 Inf 无效"
                      }
                      frame True {
                        # "报警限值有效"
                        n173 = Max & Min(x=w282, y=w277) -> (max(x,y)=w281:dbl)  [unwired: 1 out]
                        n174 = Max & Min(x=w279, y=w280) -> (min(x,y)=w278:dbl)  [unwired: 1 out]
                      }
                    }
                    n175 = Bundle(w167, w168) -> (w227:cluster{timestamp[], dbl[]})  [unwired: 1 in]
                    n176 = Bundle(w191, w192) -> (w173:cluster{timestamp[], dbl[]})  [unwired: 1 in]
                    n177 = Greater?(x=w144, y=w143) -> (0:w142:bool)
                    n178 = Subtract(x=w144, y=w209) -> (x-y=w219:dbl)
                    n179 = Multiply(x=w219, y=0.1) -> (x*y=w216:dbl)
                    n180 = Subtract(x=w171, y=w240) -> (x-y=w238:dbl)
                    n181 = Subtract(x=w161, y=w240) -> (x-y=w239:dbl)
                    n182 = Add(x=w144, y=w216) -> (x+y=w217:dbl)
                    n183 = Subtract(x=w209, y=w216) -> (x-y=w212:dbl)
                    n184 = property on="属性节点" class="XY图 (严格)"(reference=w140, "Active Plot"=w226, "Plot.Visible?"=w142) -> (error out=w221:errorcluster)  [unwired: 1 in, 1 out]
                    n185 = Less Or Equal To 0?(x=w212) -> (x <= 0?=w215:bool)
                    n186 = Select(t=0.0, s=w215, f=w212) -> (s? t:f=w213:dbl)
                    n187 = property on="属性节点" class="XYGraph (严格)"(reference=w140, error in=w221, "XScale.Maximum"=w239, "XScale.Minimum"=w238, "YScale.Maximum"=w217, "YScale.Minimum"=w213) -> ()  [unwired: 2 out]
                    n188 = in-place-match #2(w141) -> (w132:cluster{timestamp[], dbl[]})
                    n189 = in-place-match #3(w227) -> (w134:cluster{timestamp[], dbl[]})
                    n190 = in-place-match #4(w173) -> (w133:cluster{timestamp[], dbl[]})
                  }
                  n191 = in-place-array #1(w132, w134, w133) -> (w124:cluster{timestamp[], dbl[]}[])  [unwired: 3 out]
                }
                n192 = property on="坐标映射信号" class="Bool (严格)"("Val(Sgnl)"=w122) -> ()  [unwired: 2 in, 2 out]
                n193 = local write "XY图"(w124) -> ()
              }
            }
            n194 = Concatenate Strings(w59, "一级限值(Sv/h)：" ("字符串"), w88) -> (→"限值1":string)
            n195 = Concatenate Strings(w56, "二级限值(Sv/h)：" ("字符串"), w86) -> (→"限值2":string)
            n196 = Greater?(x=w70, y=w69) -> (0:w71:bool)
            n197 = case shown="真" w71 {
              tunnel: w70 -> [w117 w120]
              tunnel: w69 -> [_ w119]
              tunnel: [w117 w118] -> w67
              frame False {
                # "uSv/h"
              }
              frame True {
                # "mSv/h"
                n198 = Divide(x=w120, y=w119) -> (x/y=w118:dbl)
              }
            }
            n199 = Select(t=" m" ("F-格式字符串"), s=w71, f=" μ" ("F-格式字符串")) -> (s? t:f=w65:string)
            n200 = Number To Fractional String(number=w67, precision (6)=i16 2 ("精度(6)")) -> (F-format string=w66:string)  [unwired: 2 in]
            n201 = property on="探头状态" class="Enum (严格)"("Val(Sgnl)"=w82) -> ()  [unwired: 2 in, 2 out]
            n202 = Concatenate Strings(w66, w65) -> (w64:string)
            n203 = Concatenate Strings("累积剂量(Sv)：" ("字符串"), w64) -> (→"累积剂量":string)
          }
          event "坐标映射信号": Value Change {
            # "数值映射"
            n204 = event-data() -> ()  [unwired: 1 in, 6 out]
            n205 = stacked-sequence {
              tunnel: [w338] -> w330
              frame #0 {
                n206 = Get Date/Time In Seconds() -> (seconds since 1Jan1904=w338:timestamp)
              }
            }
            n207 = Unbundle(w326) -> (w327:timestamp[], w328:dbl[])
            n208 = property on="数值" class="Str"() -> ("Visible"=w333:bool)  [unwired: 2 in, 2 out]
            n209 = Empty Array?(array=w328) -> (empty?=w329:bool)
            n210 = Not(x=w329) -> (.not. x?=w334:bool)
            n211 = And(x=w334, y=w333) -> (x .and. y?=w332:bool)
            n212 = case shown="真" w332 {
              tunnel: w327 -> [_ w360]
              tunnel: w328 -> [_ w359]
              tunnel: w330 -> [w339 w353]
              tunnel: [w339 w353] -> w331
              frame False {
                # "空数组，或悬浮数值不可见"
              }
              frame True {
                w370 = 1000.0 ("y")
                # "非空数组，且悬数值可见"
                n213 = control-ref of="XY图"() -> (w351:refnum<vi>)
                n214 = Unbundle By Name("鼠标坐标") -> ("Horizontal"=w341:i32, "Vertical"=w340:i32)
                n215 = invoke on="调用节点" class="XY图 (严格)" method="Map Coords To XY"(reference=w351, "Coords"="鼠标坐标") -> ("XY"=w372:cluster{"X":dbl, "Y":dbl})  [unwired: 5 in, 6 out]
                n216 = property on="数值" class="Str"() -> (error out=w355:errorcluster, "Bounds"=w354:T8)  [unwired: 2 in, 1 out]
                n217 = Unbundle By Name(w354) -> ("Width"=w345:u32, "Height"=w344:u32)
                n218 = Unbundle By Name(w372) -> ("X"=w365:dbl)
                n219 = Subtract(x=w360, y=timestamp(0 s since 1904-01-01)) -> (x-y=w363:dbl[])
                n220 = Divide(x=w345, y=u32 2) -> (x/y=w347:dbl)
                n221 = call "快速逼近索引法.vi"("数值"=w365, "数组"=w363) -> ("最近索引"=w362:i32)  [unwired: 9 in]
                n222 = Subtract(x=w341, y=w347) -> (x-y=w343:dbl)
                n223 = Index Array(array=w359, index=w362) -> (element=w361:dbl)
                n224 = Subtract(x=w340, y=w344) -> (x-y=w348:u32)
                n225 = Subtract(x=w348, y=u32 10) -> (x-y=w342:u32)
                n226 = Greater Or Equal?(x=w361, y=w370) -> (x >= y?=w371:bool)
                n227 = case shown="假" w371 {
                  tunnel: w361 -> [w374 w378]
                  tunnel: w370 -> [_ w377]
                  tunnel: [w374 w376] -> w368
                  tunnel: [" μSv/h" " mSv/h"] -> w366
                  frame False {
                    # "mSv/h"
                  }
                  frame True {
                    # "uSv/h"
                    n228 = Divide(x=w378, y=w377) -> (x/y=w376:dbl)
                  }
                }
                n229 = Bundle By Name(cluster=T6 {"Left"=0, "Top"=0} ("位置"), "Left"=w343, "Top"=w342) -> (w357:T6)
                n230 = property on="数值" class="Str"(error in=w355, "Position"=w357) -> ()  [unwired: 1 in, 2 out]
                n231 = Number To Fractional String(number=w368, precision (6)=i16 2 ("精度(6)")) -> (F-format string=w367:string)  [unwired: 2 in]
                n232 = Concatenate Strings(w367, w366) -> (→"数值":string)
                n233 = Wait (ms)(milliseconds to wait=u32 30 ("等待时间（毫秒）")) -> ()  [unwired: 1 out]
              }
            }
            n234 = stacked-sequence {
              tunnel: w331 -> [w336]
              frame #0 {
                # "净处理时间为\n最少 3μs\n300点满数组 5~20ms"
                n235 = Get Date/Time In Seconds() -> (seconds since 1Jan1904=w337:timestamp)
                n236 = Subtract(x=w337, y=w336) -> (x-y=→"计算时间":dbl)
              }
            }
          }
          event "XY图": Mouse Enter {
            w379 = TRUE  # T
            # "进入，显示"
            # "显示悬浮数值"
            n237 = event-data() -> ()  [unwired: 1 in, 4 out]
            n238 = property on="数值" class="Str"("Visible"=w379) -> ()  [unwired: 2 in, 2 out]
          }
          event "XY图": Mouse Leave {
            w381 = FALSE  # F
            # "离开，隐藏"
            # "隐藏悬浮数值"
            n239 = event-data() -> ()  [unwired: 1 in, 4 out]
            n240 = property on="数值" class="Str"("Visible"=w381) -> ()  [unwired: 2 in, 2 out]
          }
          event "XY图": Mouse Move {
            # "触发数值映射事件"
            n241 = event-data() -> ("Coords"=w383:T1)  [unwired: 1 in, 4 out]
            n242 = flat-sequence {
              tunnel: w383 -> [w385]
              frame #0 {
                n243 = local write "鼠标坐标"(w385) -> ()
              }
              frame #1 {
                n244 = property on="坐标映射信号" class="Bool (严格)"("Val(Sgnl)"=FALSE ("值(信号)")) -> ()  [unwired: 2 in, 2 out]
              }
            }
          }
        }
      }
    }
  }
